vi "Panel Create Message Queue.vi"(8 "error in (no error)":errorcluster, 11 "Panel Control_Ref in":refnum<class "Panel Controller.lvclass">) -> (0 "error out":errorcluster, 3 "Panel Control_Ref out":refnum<class "Panel Controller.lvclass">)   [LabVIEW 2015, in "Panel Controller.lvclass"]
uses:
  Panel Controller.lvclass
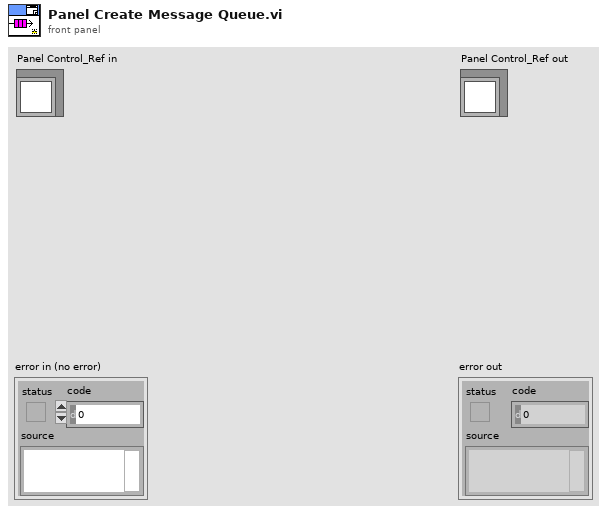
[diagram p1: front panel]
types:
  T1 = typedef "Panel Controller.lvclass/ObjectAttributes.ctl" = cluster{"Sub Panel Ref":refnum<vi>, "Panel_Q":refnum<queue>, "VI Running Refnum":refnum<vi>, "Brower Controller_Q":refnum<class "Message Enqueuer.lvclass">, "GUI Control Builder Director.lvclass":refnum<class "GUI Control Builder Director.lvclass">, "Panel GUI Manager.lvclass":refnum<class "Panel GUI Manager.lvclass">}
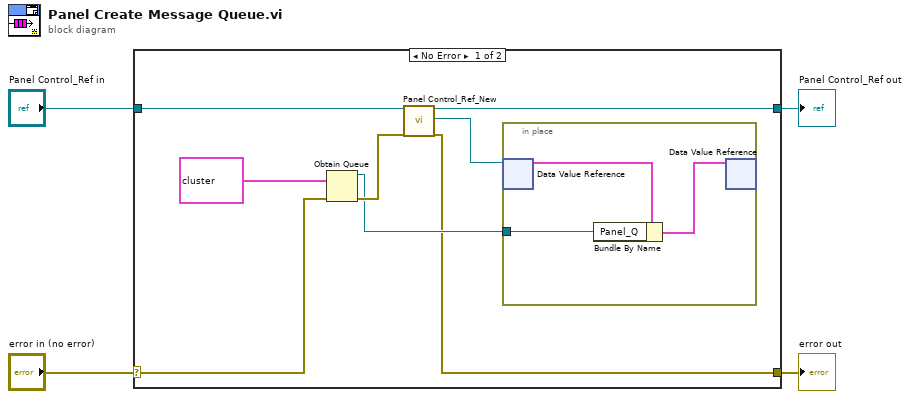
[diagram p0: block diagram]
diagram:
  n1 = case shown="No Error" "error in (no error)" {
    selector: "error in (no error)" -> [w11 w17]
    tunnel: [w5 w17] -> w3
    tunnel: [w6 w16] -> w1
    tunnel: "Panel Control_Ref in" -> [w10 w16]
    frame No Error {
      n2 = Obtain Queue(element data type=cluster{"Data":variant, "Msg":string} {"Data"=variant, "Msg"=""}, error in (no error)=w11) -> (queue out=w7:refnum<queue>, error out=w9:errorcluster)  [unwired: 3 in, 1 out]
      n3 = call "Panel Control_Ref_New.vi"("reference in"=w10, "error in (no error)"=w9) -> ("reference out"=w6:refnum<class "Panel Controller.lvclass">, "DVRRefOut"=w8:refnum<data-value>, "error out"=w5:errorcluster)  [unwired: 14 in, 1 out]
      n4 = in-place {
        in-place-border: w7 -> [w14]
        n5 = in-place-dvr #1(w8) -> (w15:T1)  [unwired: 1 out]
        n6 = Bundle By Name(cluster=w15, "Panel_Q"=w14) -> (w13:T1)
        n7 = in-place-dvr #1(w13) -> ()  [unwired: 2 out]
      }
    }
    frame Error {
    }
  }
  "error out" <- w3
  "Panel Control_Ref out" <- w1
